vi "Current Ramp Act.vi"(0 "command text in":string[](array[string])) -> ()   [LabVIEW 2020]
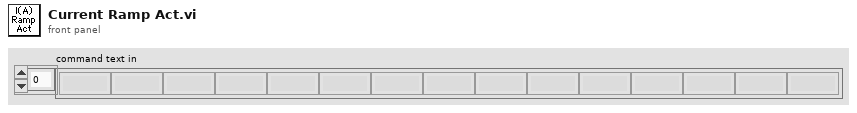
[diagram p1: front panel]
types:
  T1 = typedef "CurrentRamp.ctl" = cluster{"VISA Resource Name":refnum<visa-resource-name>, "extra wait":i32, "start":dbl, "end":dbl, "Sweep Time (H:M:S)":dbl, "Log Linear":bool, "interval(sec)":dbl, "Select Instrument":T2}
  T2 = typedef "CurrentRamp Instrument.ctl" = enum16{"Keithley 6221 Coarse"}
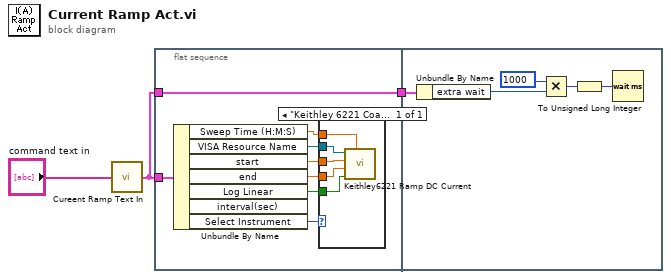
[diagram p0: block diagram]
diagram:
  n1 = call "Cureent Ramp Text In.vi"("command text in"="command text in") -> ("Current Ramp"=w2:T1)
  n2 = flat-sequence {
    tunnel: w2 -> [w10]
    tunnel: w2 -> [w11]
    tunnel: [w11] -> w1
    tunnel: w1 -> [w18]
    frame #0 {
      n3 = Unbundle By Name(w10) -> ("Sweep Time (H:M:S)"=w9:dbl, "VISA Resource Name"=w8:refnum<visa-resource-name>, "start"=w7:dbl, "end"=w6:dbl, "Log Linear"=w5:bool, "Select Instrument"=w4:T2)  [unwired: 1 out]
      n4 = case shown="\"Keithley 6221 Coarse\", Default" w4 {
        tunnel: w9 -> [w16]
        tunnel: w8 -> [w15]
        tunnel: w7 -> [w14]
        tunnel: w6 -> [w13]
        tunnel: w5 -> [w12]
        frame "Keithley 6221 Coarse", Default {
          n5 = call "Keithley6221 Ramp DC Current.vi"("Sweep Time (H:M:S)"=w16, "Mapping"=w12, "End Current (A)"=w13, "Start Current (A)"=w14, "K6221 GPIB address"=w15) -> ()  [unwired: 6 in, 1 out]
        }
      }
    }
    frame #1 {
      n6 = Unbundle By Name(w18) -> ("extra wait"=w17:i32)
      n7 = Multiply(x=1000 ("y"), y=w17) -> (x*y=w20:i32)
      n8 = To Unsigned Long Integer(number=w20) -> (unsigned 32bit integer=w19:u32)
      n9 = Wait (ms)(milliseconds to wait=w19) -> ()  [unwired: 1 out]
    }
  }
